vi "ROC Plot.vi"(10 "Sens.":dbl[](array[numeric])=[0.111111111, 0.222222222, 0.333333333, 0.444444444, 0.444444444, 0.555555556, 0.666666667, 0.666666667, 0.666666667, 0.777777778, 0.777777778, 0.777777778, 0.777777778, 0.777777778, 0.888888889, 0.888888889, 1.0, 1.0], 11 "1-Spec.":dbl[](array[numeric])=[0.0, 0.0, 0.0, 0.0, 0.111111111, 0.111111111, 0.111111111, 0.222222222, 0.333333333, 0.333333333, 0.444444444, 0.555555556, 0.666666667, 0.777777778, 0.777777778, 0.888888889, 0.888888889, 1.0]) -> ()   [LabVIEW 2020]
uses:
  <vilib>/Heliosphere Research LLC/Advanced Plotting Toolkit/Advanced Plotting Toolkit.lvlib
panel:
  out "AUC":dbl
  out "Picture":picture
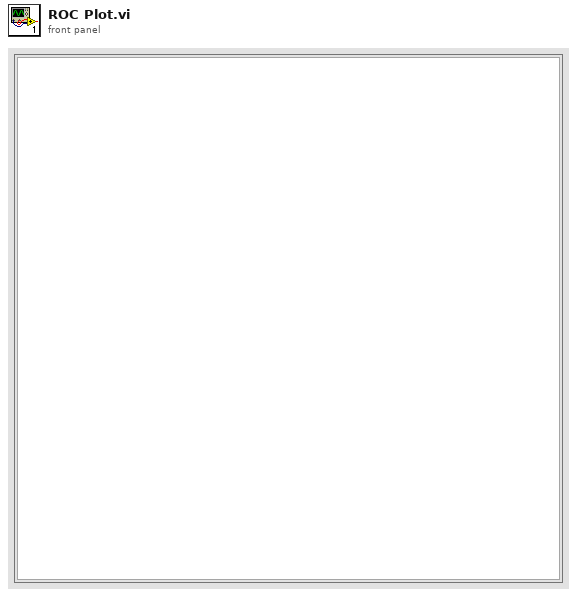
[diagram p1: front panel]
types:
  T1 = typedef "Advanced Plotting Toolkit.lvlib/PlotID.ctl" = i32
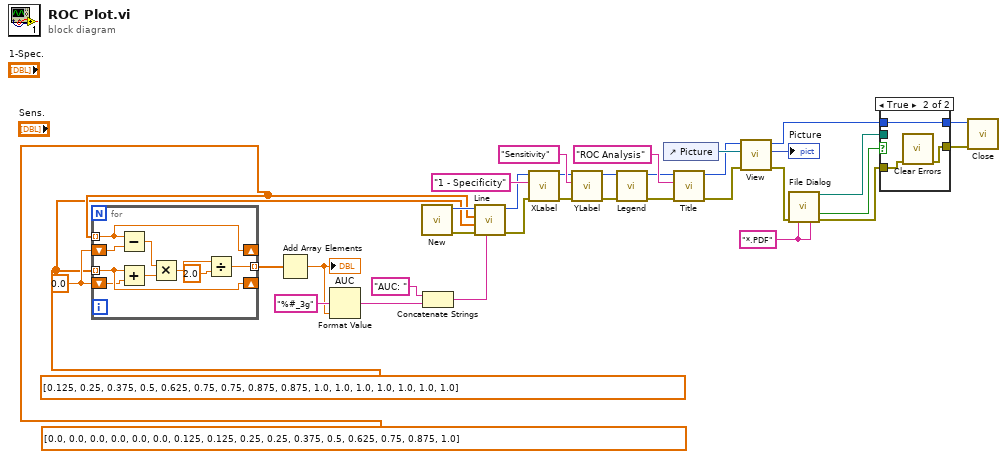
[diagram p0: block diagram]
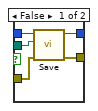
[diagram p2: hidden frame]
diagram:
  w2 = dbl[] [0.0, 0.0, 0.0, 0.0, 0.0, 0.0, 0.125, 0.125, 0.25, 0.25, 0.375, 0.5, 0.625, 0.75, 0.875, 1.0] ("1-Spec.")
  w1 = dbl[] [0.125, 0.25, 0.375, 0.5, 0.625, 0.75, 0.75, 0.875, 0.875, 1.0, 1.0, 1.0, 1.0, 1.0, 1.0, 1.0] ("1-Spec.")
  w9 = "*.PDF" ("pattern (all files)")
  w23 = 0.0
  n1 = for {
    tunnel: w2 -> [w38] mode=indexing
    tunnel: w1 -> [w37] mode=indexing
    tunnel: [w42] -> w24 mode=indexing
    shift-right: [w38] -> _
    shift-left: w23 -> [w39]
    shift-right: [w37] -> _
    shift-left: w23 -> [w36]
    n2 = Subtract(x=w38, y=w39) -> (x-y=w40:dbl)
    n3 = Add(x=w37, y=w36) -> (x+y=w35:dbl)
    n4 = Multiply(x=w40, y=w35) -> (x*y=w43:dbl)
    n5 = Divide(x=w43, y=2.0) -> (x/y=w42:dbl)
  }
  n6 = Add Array Elements(numeric array=w24) -> (sum=w13:dbl)
  "AUC" <- w13
  n7 = Format Value(format string="%#_3g" ("string (\"\")"), value (0)=w13) -> (output string=w12:string)  [unwired: 1 in]
  n8 = call <vilib>:"New.vi"() -> ("error out"=w34:errorcluster, "Plot ID"=w29:T1)  [unwired: 10 in]
  n9 = Concatenate Strings("AUC: " ("string"), w12) -> (w15:string)
  n10 = call <vilib>:"Line.vi"("Legend Title"=w15, "error in (no error)"=w34, "Y Data"=w1, "X Data"=w2, "Plot ID"=w29) -> ("error out"=w30:errorcluster, "Plot ID out"=w28:T1)  [unwired: 5 in]
  n11 = call <vilib>:"XLabel.vi"("error in (no error)"=w30, "Label"="1 - Specificity", "Plot ID"=w28) -> ("error out"=w31:errorcluster, "Plot ID out"=w27:T1)  [unwired: 7 in]
  n12 = call <vilib>:"YLabel.vi"("error in (no error)"=w31, "Label"="Sensitivity", "Plot ID"=w27) -> ("error out"=w21:errorcluster, "Plot ID out"=w22:T1)  [unwired: 7 in]
  n13 = call <vilib>:"Legend.vi"("error in (no error)"=w21, "Plot ID"=w22) -> ("error out"=w18:errorcluster, "Plot ID Out"=w19:T1)  [unwired: 8 in]
  n14 = control-ref of="Picture"() -> (w25:refnum<vi>)
  n15 = call <vilib>:"Title.vi"("error in (no error)"=w18, "Title"="ROC Analysis", "Plot ID"=w19) -> ("error out"=w17:errorcluster, "Plot ID out"=w16:T1)  [unwired: 7 in]
  n16 = call <vilib>:"View.vi"("error in (no error)"=w17, "Ref for Sizing"=w25, "Plot ID"=w16) -> ("error out"=w10:errorcluster, "Picture"=→"Picture":picture, "Plot ID Out"=w7:T1)  [unwired: 6 in]
  n17 = call "File Dialog"("error in"=w10, "pattern (all files)"=w9, "pattern label"=w9) -> ("selected path"=w4:path, "cancelled"=w3:bool, "error out"=w8:errorcluster)  [unwired: 9 in, 1 out]
  n18 = case shown="True" w3 {
    tunnel: w8 -> [w48 w50]
    tunnel: w7 -> [w47 w51]
    tunnel: [w46 w51] -> w6
    tunnel: [w45 w49] -> w5
    tunnel: w4 -> [w44 _]
    frame False {
      n19 = call <vilib>:"Save.vi"("error in (no error)"=w48, "Path"=w44, "Plot ID In"=w47) -> ("error out"=w45:errorcluster, "Plot ID Out"=w46:T1)  [unwired: 7 in]
    }
    frame True {
      n20 = call <vilib>:"Clear Errors.vi"("error in (no error)"=w50) -> ("error out"=w49:errorcluster)  [unwired: 5 in, 1 out]
    }
  }
  n21 = call <vilib>:"Close.vi"("error in (no error)"=w5, "Plot ID"=w6) -> ()  [unwired: 9 in, 1 out]
